vi "KeyDown.vi"(8 "error in (no error)":errorcluster, 10 "Char":i16, 11 "View in":refnum<class "View.lvclass">) -> (0 "error out":errorcluster, 3 "View out":refnum<class "View.lvclass">)   [LabVIEW 2024, in "GUI.lvlib" / "View.lvclass"]
uses:
  View.lvclass
  View.lvclass/View.ctl
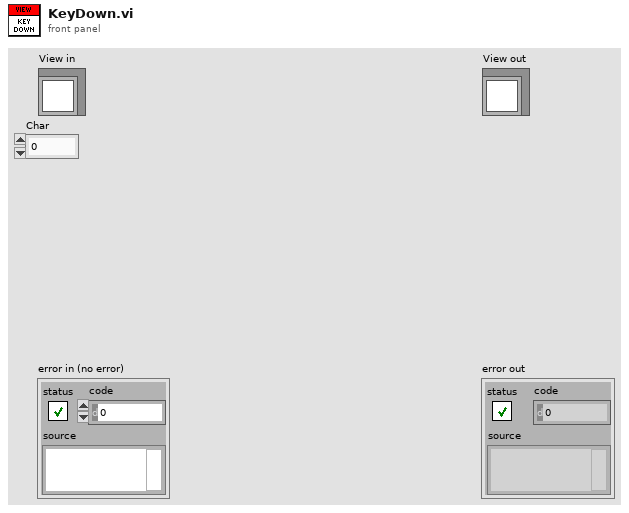
[diagram p1: front panel]
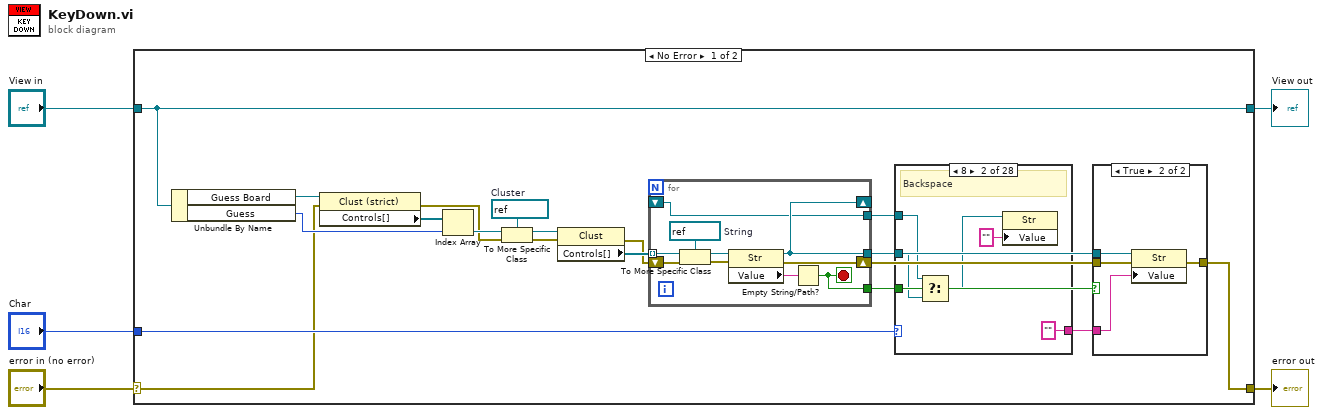
[diagram p0: block diagram]
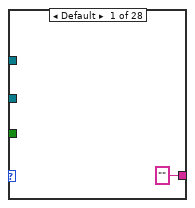
[diagram p3: hidden frame]
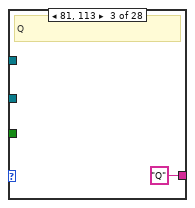
[diagram p4: hidden frame]
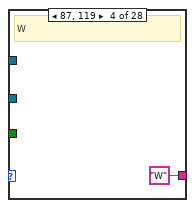
[diagram p5: hidden frame]
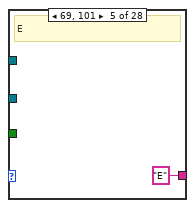
[diagram p6: hidden frame]
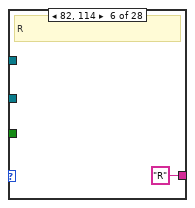
[diagram p7: hidden frame]
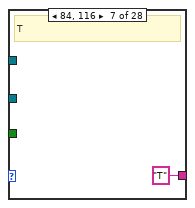
[diagram p8: hidden frame]
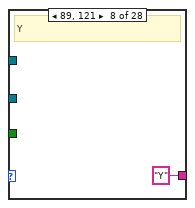
[diagram p9: hidden frame]
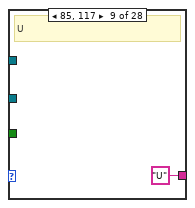
[diagram p10: hidden frame]
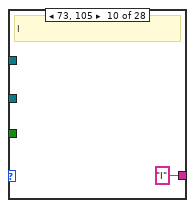
[diagram p11: hidden frame]
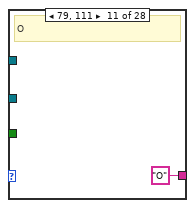
[diagram p12: hidden frame]
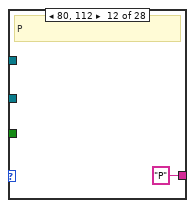
[diagram p13: hidden frame]
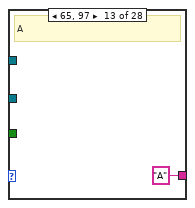
[diagram p14: hidden frame]
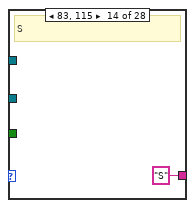
[diagram p15: hidden frame]
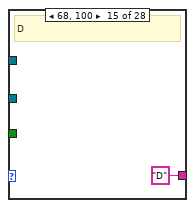
[diagram p16: hidden frame]
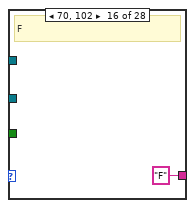
[diagram p17: hidden frame]
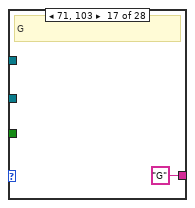
[diagram p18: hidden frame]
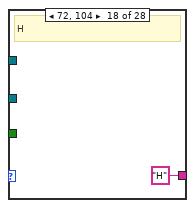
[diagram p19: hidden frame]
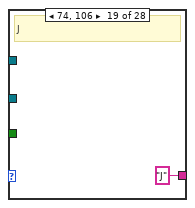
[diagram p20: hidden frame]
diagram:
  n1 = case shown="No Error" "error in (no error)" {
    selector: "error in (no error)" -> [w12 w74]
    tunnel: [w9 w74] -> w4
    tunnel: [w23 w73] -> w2
    tunnel: "View in" -> [w23 w73]
    tunnel: "Char" -> [w24 _]
    frame No Error {
      w18 = refnum<vi> refnum  # Cluster
      n2 = Unbundle By Name(w23) -> ("Guess Board"=w22:refnum<vi>, "Guess"=w20:i32)
      n3 = property class="Clust (strict)"(reference=w22, error in=w12) -> (error out=w14:errorcluster, "Controls[]"=w21:refnum<vi>[])  [unwired: 1 out]
      n4 = Index Array(array=w21, index=w20) -> (element=w19:refnum<vi>)
      n5 = To More Specific Class(target class=w18, reference=w19, error in=w14) -> (specific class reference=w17:refnum<vi>, error out=w13:errorcluster)
      n6 = property class="Clust"(reference=w17, error in=w13) -> (error out=w11:errorcluster, "Controls[]"=w16:refnum<vi>[])  [unwired: 1 out]
      n7 = for {
        tunnel: w16 -> [w38] mode=indexing
        tunnel: [w32] -> w6
        shift-right: [w35] -> w10
        shift-left: w11 -> [w34]
        shift-right: [w32] -> _
        shift-left: _ -> [w31]
        tunnel: [w31] -> w8
        tunnel: [w30] -> w7
        stop <- w30 stop-if-true
        w39 = refnum<vi> refnum  # String
        n8 = To More Specific Class(target class=w39, reference=w38, error in=w34) -> (specific class reference=w37:refnum<vi>, error out=w33:errorcluster)
        n9 = property class="Str"(reference=w37, error in=w33) -> (reference out=w32:refnum<vi>, error out=w35:errorcluster, "Value"=w36:string)
        n10 = Empty String/Path?(string/path=w36) -> (empty?=w30:bool)
      }
      n11 = case shown="8" w24 {
        tunnel: ["" "" "Q" "W" "E" "R" "T" "Y" "U" "I" "O" "P" "A" "S" "D" "F" "G" "H" "J" "K" "L" "Z" "X" "C" "V" "B" "N" "M"] -> w15
        tunnel: w8 -> [_ w43 _ _ _ _ _ _ _ _ _ _ _ _ _ _ _ _ _ _ _ _ _ _ _ _ _ _]
        tunnel: w7 -> [_ w44 _ _ _ _ _ _ _ _ _ _ _ _ _ _ _ _ _ _ _ _ _ _ _ _ _ _]
        tunnel: w6 -> [_ w41 _ _ _ _ _ _ _ _ _ _ _ _ _ _ _ _ _ _ _ _ _ _ _ _ _ _]
        frame Default {
        }
        frame 8 {
          # "Backspace"
          n12 = Select(t=w43, s=w44, f=w41) -> (s? t:f=w42:refnum<vi>)
          n13 = property class="Str"(reference=w42, "Value"="") -> ()  [unwired: 1 in, 2 out]
        }
        frame 81, 113 {
          # "Q"
        }
        frame 87, 119 {
          # "W"
        }
        frame 69, 101 {
          # "E"
        }
        frame 82, 114 {
          # "R"
        }
        frame 84, 116 {
          # "T"
        }
        frame 89, 121 {
          # "Y"
        }
        frame 85, 117 {
          # "U"
        }
        frame 73, 105 {
          # "I"
        }
        frame 79, 111 {
          # "O"
        }
        frame 80, 112 {
          # "P"
        }
        frame 65, 97 {
          # "A"
        }
        frame 83, 115 {
          # "S"
        }
        frame 68, 100 {
          # "D"
        }
        frame 70, 102 {
          # "F"
        }
        frame 71, 103 {
          # "G"
        }
        frame 72, 104 {
          # "H"
        }
        frame 74, 106 {
          # "J"
        }
        frame 75, 107 {
          # "K"
        }
        frame 76, 108 {
          # "L"
        }
        frame 90, 122 {
          # "Z"
        }
        frame 88, 120 {
          # "X"
        }
        frame 67, 99 {
          # "C"
        }
        frame 86, 118 {
          # "V"
        }
        frame 66, 98 {
          # "B"
        }
        frame 78, 110 {
          # "N"
        }
        frame 77, 109 {
          # "M"
        }
      }
      n14 = case shown="True" w7 {
        tunnel: w6 -> [_ w29]
        tunnel: w15 -> [_ w28]
        tunnel: w10 -> [w25 w27]
        tunnel: [w25 w26] -> w9
        frame False {
        }
        frame True {
          n15 = property class="Str"(reference=w29, error in=w27, "Value"=w28) -> (error out=w26:errorcluster)  [unwired: 1 out]
        }
      }
    }
    frame Error {
    }
  }
  "error out" <- w4
  "View out" <- w2
